vi "Camera Finish.vi"   [LabVIEW 2013]
types:
  T1 = typedef "WPI_ServoDeviceRef.ctl" = cluster{"DeviceStatus":errorcluster, "Digital Module":T2, "PWM Channel":T3, "DeadBand":T4}
  T2 = typedef "FPGA_TypedefDigitalModule.ctl" = enum16{"Digital Module 1", "Digital Module 2"}
  T3 = typedef "FPGA_DIOPWMChannel.ctl" = enum8{"PWM 1", "PWM 2", "PWM 3", "PWM 4", "PWM 5", "PWM 6", "PWM 7", "PWM 8", "PWM 9", "PWM 10", "Invalid"}
  T4 = typedef "WPI_PWMDeadband.ctl" = cluster{"Name":string, "maxPositivePwm":i32, "minPositivePwm":i32, "centerPwm":i32, "maxNegativePwm":i32, "minNegativePwm":i32, "angularRange":u16}
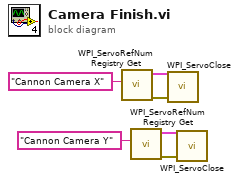
[diagram p0: block diagram]
diagram:
  n1 = call <vilib>:"WPI_ServoRefNum Registry Get.vi"("refnum name"="Cannon Camera X") -> ("error out"=w6:errorcluster, "ServoDeviceRef"=w5:T1)  [unwired: 9 in]
  n2 = call <vilib>:"WPI_ServoRefNum Registry Get.vi"("refnum name"="Cannon Camera Y") -> ("error out"=w1:errorcluster, "ServoDeviceRef"=w2:T1)  [unwired: 9 in]
  n3 = call <vilib>:"WPI_ServoClose.vi"("error in (no error)"=w6, "MotorControlDevRef"=w5) -> ()  [unwired: 9 in, 1 out]
  n4 = call <vilib>:"WPI_ServoClose.vi"("error in (no error)"=w1, "MotorControlDevRef"=w2) -> ()  [unwired: 9 in, 1 out]
